vi "Plugin - Current Time.vi"() -> ()   [LabVIEW 2014]
doc: "現在の時刻を表示するサブパネルプラグインVI。"
panel:
  in  "パラメータ":string[](array[string])
  out "現在の時間":string
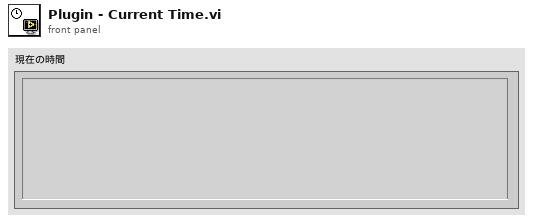
[diagram p1: front panel]
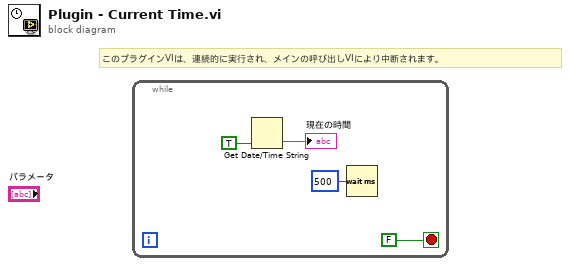
[diagram p0: block diagram]
diagram:
  # "このプラグインVIは、連続的に実行され、メインの呼び出しVIにより中断されます。"
  n1 = while {
    stop <- FALSE stop-if-true
    n2 = Get Date/Time String(want seconds? (F)=TRUE) -> (time string=→"現在の時間":string)  [unwired: 2 in, 1 out]
    n3 = Wait (ms)(milliseconds to wait=u32 500) -> ()  [unwired: 1 out]
  }
